vi "Client 1 Cluster.vi"() -> (0 "Cluster":T1)   [LabVIEW 2009]
doc: "Cluster for the Cliens in the QDMH Client-Server demonstration.\n\nAAL 9/09"
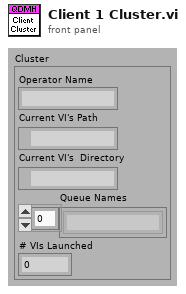
[diagram p1: front panel]
types:
  T1 = cluster{"Operator Name":string, "Current VI's Path":path, "Current VI's  Directory":path, "Queue Names":string[], "# VIs Launched":i32}
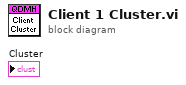
[diagram p0: block diagram]
diagram:
